vi "HEWH Update Power Display.vi"(10 "Water Heater GEA2 Data":T2 {"Hyperterminal Data"."CRC" format="%x"; "Hyperterminal Data"."Length" format="%x"; "Hyperterminal Data"."Command" format="%x"; "Hyperterminal Data"."Destination" format="%x"; "Hyperterminal Data"."Source" format="%x"}, 11 "POWER DAQ LOOP in":T1) -> (3 "POWER DAQ LOOP out":T1)   [LabVIEW 2019]
uses:
  Utility/GEA2 Commands/HEWH/Type Definitions/GEA2 Commands WaterHeater GEA2 Data.ctl
  Utility/GEA2 Commands/HEWH/Type Definitions/GEA2 Commands Button Status.ctl
  Utility/GEA2 Commands/HEWH/Type Definitions/GEA2 Commands Status Query.ctl
  Utility/GEA2 Commands/HEWH/Type Definitions/GEA2 Commands Service Error Codes.ctl
  Type Definitions/HEWH Power Elements.ctl
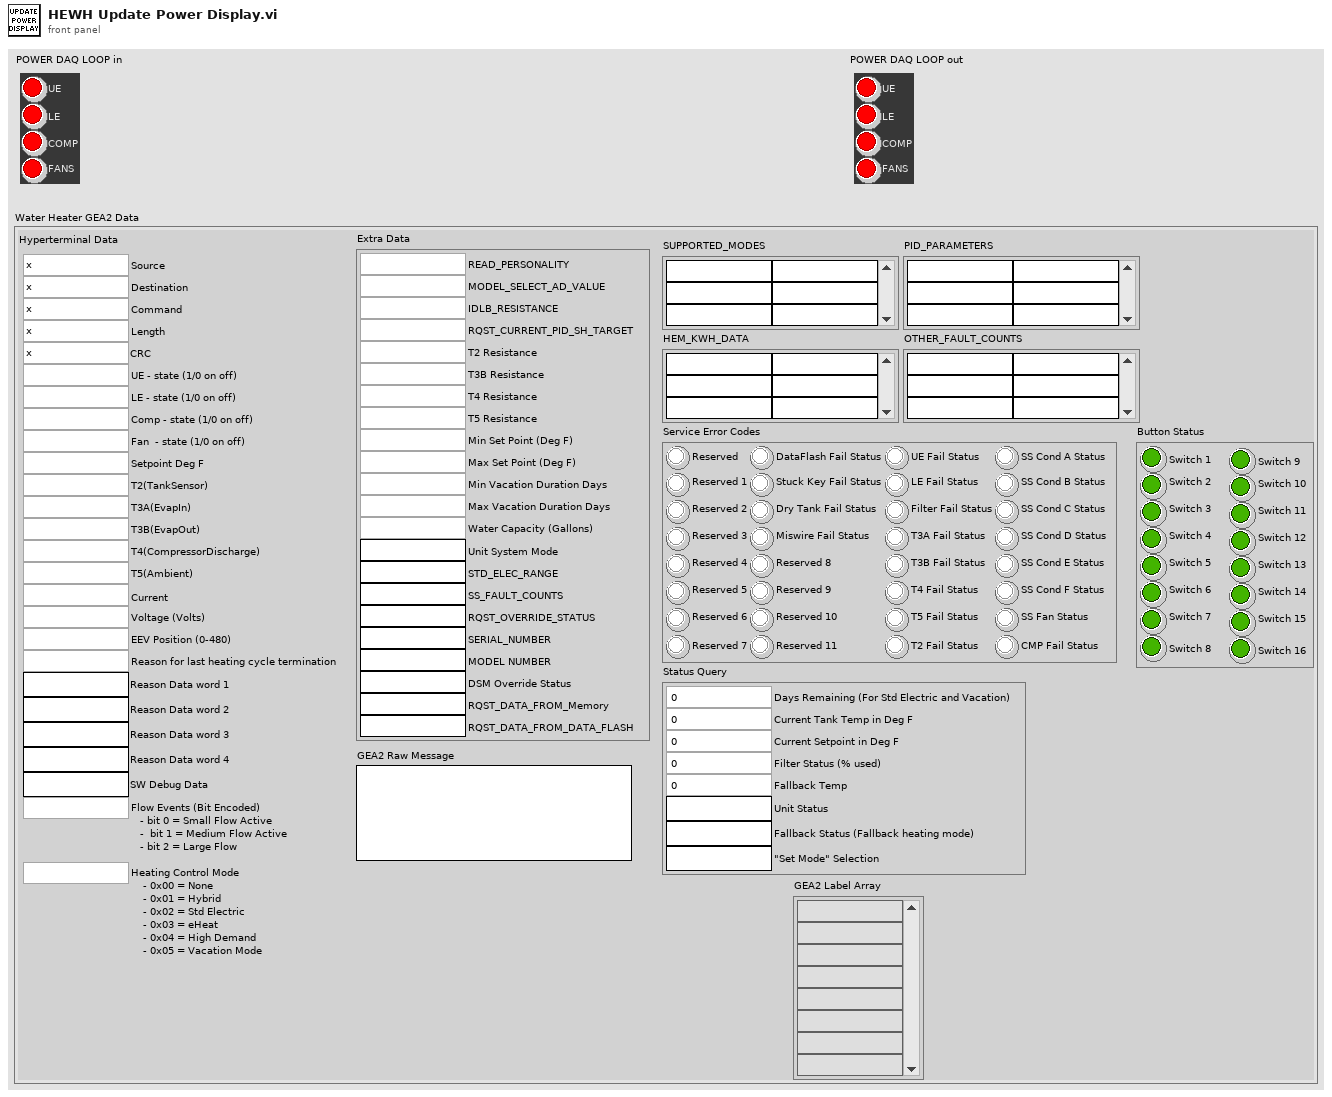
[diagram p1: front panel]
types:
  T1 = typedef "HEWH Power Elements.ctl" = cluster{"UE":bool, "LE":bool, "COMP":bool, "FANS":bool}
  T2 = typedef "GEA2 Commands WaterHeater GEA2 Data.ctl" = cluster{"GEA2 Label Array":string[], "PID_PARAMETERS":string[][], "SUPPORTED_MODES":string[][], "Button Status":T3, "Status Query":T4, "Service Error Codes":T5, "HEM_KWH_DATA":string[][], "OTHER_FAULT_COUNTS":string[][], "GEA2 Raw Message":string, "Hyperterminal Data":cluster{"Source":u8, "Destination":u8, "Command":u8, "Length":u8, "CRC":u16, "UE - state (1/0 on off)":u8, "LE - state (1/0 on off)":u8, "Comp - state (1/0 on off)":u8, "Fan  - state (1/0 on off)":u8, "Setpoint Deg F":i32, "T2(TankSensor)":dbl, "T3A(EvapIn)":dbl, "T3B(EvapOut)":dbl, "T4(CompressorDischarge)":dbl, "T5(Ambient)":dbl, "Current":dbl, "Voltage (Volts)":u16, "EEV Position (0-480)":u16, "Reason for last heating cycle termination":u16, "Reason Data word 1":string, "Reason Data word 2":string, "Reason Data word 3":string, "Reason Data word 4":string, "SW Debug Data":string, "Flow Events (Bit Encoded)":u16, "Heating Control Mode":u16}, "Extra Data":cluster{"Water Capacity (Gallons)":u32, "Max Vacation Duration Days":u32, "Min Vacation Duration Days":u32, "Max Set Point (Deg F)":u32, "Min Set Point (Deg F)":u32, "T5 Resistance":u32, "T4 Resistance":u32, "T3B Resistance":u32, "T2 Resistance":u32, "STD_ELEC_RANGE":string, "SS_FAULT_COUNTS":string, "SERIAL_NUMBER":string, "READ_PERSONALITY":u8, "RQST_OVERRIDE_STATUS":string, "MODEL_SELECT_AD_VALUE":u32, "MODEL NUMBER":string, "IDLB_RESISTANCE":u32, "DSM Override Status":string, "RQST_DATA_FROM_Memory":string, "RQST_DATA_FROM_DATA_FLASH":string, "RQST_CURRENT_PID_SH_TARGET":u16, "Unit System Mode":string}}
  T3 = typedef "GEA2 Commands Button Status.ctl" = cluster{"Switch 1":bool, "Switch 2":bool, "Switch 3":bool, "Switch 4":bool, "Switch 5":bool, "Switch 6":bool, "Switch 7":bool, "Switch 8":bool, "Switch 9":bool, "Switch 10":bool, "Switch 11":bool, "Switch 12":bool, "Switch 13":bool, "Switch 14":bool, "Switch 15":bool, "Switch 16":bool}
  T4 = typedef "GEA2 Commands Status Query.ctl" = cluster{"Days Remaining (For Std Electric and Vacation)":u8, "Unit Status":string, "Current Tank Temp in Deg F":u8, "Current Setpoint in Deg F":u8, "Filter Status (% used)":u8, "Fallback Status (Fallback heating mode)":string, "Fallback Temp":u8, "\"Set Mode\" Selection":string}
  T5 = typedef "GEA2 Commands Service Error Codes.ctl" = cluster{"Reserved":bool, "Reserved 1":bool, "Reserved 2":bool, "Reserved 3":bool, "Reserved 4":bool, "Reserved 5":bool, "Reserved 6":bool, "Reserved 7":bool, "DataFlash Fail Status":bool, "Stuck Key Fail Status":bool, "Dry Tank Fail Status":bool, "Miswire Fail Status":bool, "Reserved 8":bool, "Reserved 9":bool, "Reserved 10":bool, "Reserved 11":bool, "UE Fail Status":bool, "LE Fail Status":bool, "Filter Fail Status":bool, "T3A Fail Status":bool, "T3B Fail Status":bool, "T4 Fail Status":bool, "T5 Fail Status":bool, "T2 Fail Status":bool, "SS Cond A Status":bool, "SS Cond B Status":bool, "SS Cond C Status":bool, "SS Cond D Status":bool, "SS Cond E Status":bool, "SS Cond F Status":bool, "SS Fan Status":bool, "CMP Fail Status":bool}
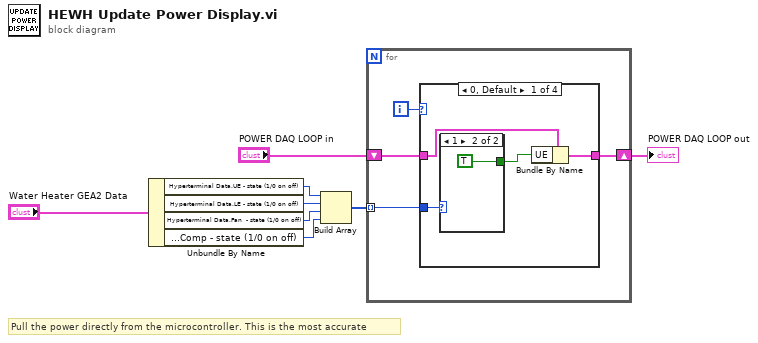
[diagram p0: block diagram]
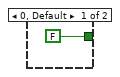
[diagram p2: hidden frame]
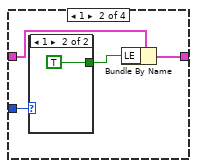
[diagram p3: hidden frame]
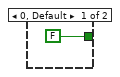
[diagram p4: hidden frame]
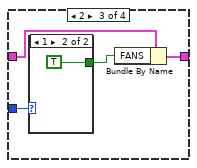
[diagram p5: hidden frame]
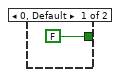
[diagram p6: hidden frame]
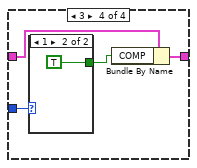
[diagram p7: hidden frame]
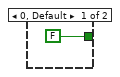
[diagram p8: hidden frame]
diagram:
  # "Pull the power directly from the microcontroller. This is the most accurate"
  n1 = Unbundle By Name("Water Heater GEA2 Data") -> ("Hyperterminal Data.UE - state (1/0 on off)"=w4:u8, "Hyperterminal Data.LE - state (1/0 on off)"=w5:u8, "Hyperterminal Data.Fan  - state (1/0 on off)"=w6:u8, "Hyperterminal Data.Comp - state (1/0 on off)"=w7:u8)
  n2 = Build Array(w4, w5, w6, w7) -> (w8:u8[])
  n3 = for {
    tunnel: w8 -> [w9] mode=indexing
    shift-right: [w11] -> w2
    shift-left: "POWER DAQ LOOP in" -> [w12]
    i -> [w10]
    n4 = case shown="0, Default" w10 {
      tunnel: w12 -> [w16 w20 w27 w33]
      tunnel: [w15 w21 w26 w32] -> w11
      tunnel: w9 -> [w14 w19 w25 w31]
      frame 0, Default {
        n5 = case shown="1" w14 {
          tunnel: [FALSE TRUE] -> w13
          frame 0, Default {
          }
          frame 1 {
          }
        }
        n6 = Bundle By Name(cluster=w16, "UE"=w13) -> (w15:T1)
      }
      frame 1 {
        n7 = case shown="1" w19 {
          tunnel: [FALSE TRUE] -> w22
          frame 0, Default {
          }
          frame 1 {
          }
        }
        n8 = Bundle By Name(cluster=w20, "LE"=w22) -> (w21:T1)
      }
      frame 2 {
        n9 = case shown="1" w25 {
          tunnel: [FALSE TRUE] -> w28
          frame 0, Default {
          }
          frame 1 {
          }
        }
        n10 = Bundle By Name(cluster=w27, "FANS"=w28) -> (w26:T1)
      }
      frame 3 {
        n11 = case shown="1" w31 {
          tunnel: [FALSE TRUE] -> w34
          frame 0, Default {
          }
          frame 1 {
          }
        }
        n12 = Bundle By Name(cluster=w33, "COMP"=w34) -> (w32:T1)
      }
    }
  }
  "POWER DAQ LOOP out" <- w2
